vi "LabJackU6_Read.vi"(8 "error in":errorcluster, 9 "Positive Channel #":i32=2, 10 "n_samples":i32=10, 11 "Handle In":i32) -> (0 "error out":errorcluster, 1 "ADC_Array":dbl[](array[numeric]), 2 "Mean ADC Voltage":dbl format="%.5f", 3 "Handle Out":i32)   [LabVIEW 2019]
uses:
  <vilib>/Analysis/baseanly.llb/Mean (DBL).vi
  <vilib>/Analysis/NI_AALBase.lvlib
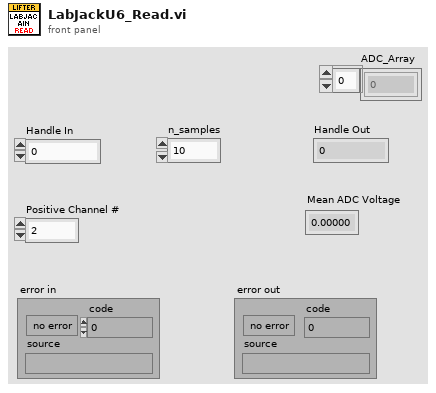
[diagram p1: front panel]
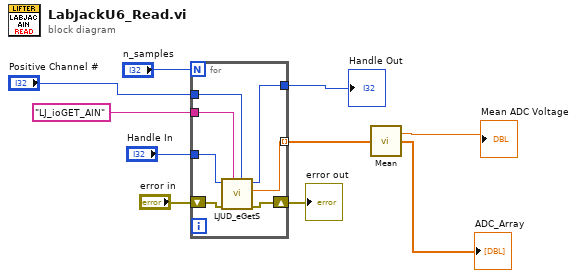
[diagram p0: block diagram]
diagram:
  n1 = for {
    N: "n_samples" -> [_]
    shift-right: [w15] -> w7
    shift-left: "error in" -> [w16]
    tunnel: "Handle In" -> [w14]
    tunnel: "LJ_ioGET_AIN" -> [w13]
    tunnel: "Positive Channel #" -> [w12]
    tunnel: [w11] -> w3
    tunnel: [w10] -> w2 mode=indexing
    n2 = call "LJUD_eGetS.vi"("Channel"=w12, "IOType"=w13, "error in"=w16, "Handle In"=w14) -> ("error out"=w15:errorcluster, "Value Read"=w10:dbl, "Handle Out"=w11:i32)  [unwired: 5 in]
  }
  "error out" <- w7
  "Handle Out" <- w3
  "ADC_Array" <- w2
  n3 = call-poly <vilib>:"Mean.vi"("X"=w2) -> ("mean"=→"Mean ADC Voltage":dbl)  [unwired: 1 out]
